vi "SC_schleife_20TVTI.vi"   [LabVIEW 2019]
uses:
  Monitors/Utility/Monitor Communication/Gustav/20TVTI_Control.ctl
  Global/Global Variables/global.vi
  Instrument_Setup.vi
  Global/Global Variables/Data_Display_global.vi
types:
  T1 = typedef "20TVTI_Cluster.ctl" = cluster{"Temperatur (K)":dbl, "Setpoint (K)":dbl, "Rate (K/min)":dbl, "Heater (%)":dbl, "NV (%)":dbl, "Heater Manual":bool, "NV Manual":bool, "Go to Set":bool, "Heater SP":dbl, "Valid?":bool, "Set Heater SP":bool, "Set NV SP":bool, "Heater (%) Display":dbl, "NV (%) Display":dbl, "NV Setpoint":dbl, "Change Heater Status":bool, "Change NV Status":bool, "Stop":bool, "Current T Setpoint":dbl, "Sweeping?":bool, "Sweep Mode":string, "Change Sweep Mode":bool}
  T2 = typedef "20TVTI_Control.ctl" = cluster{"Set VTI SP":bool, "Change NV Status":bool, "Set NV Setpoint":bool, "Change Heater Status":bool, "Set Heater Setpoint":bool, "Stop Sweep":bool, "Setpoint (K)":dbl, "Rate (K/min)":dbl, "Setpoint Heater":dbl, "Setpoint NV":dbl, "Change Sweep Mode":bool}
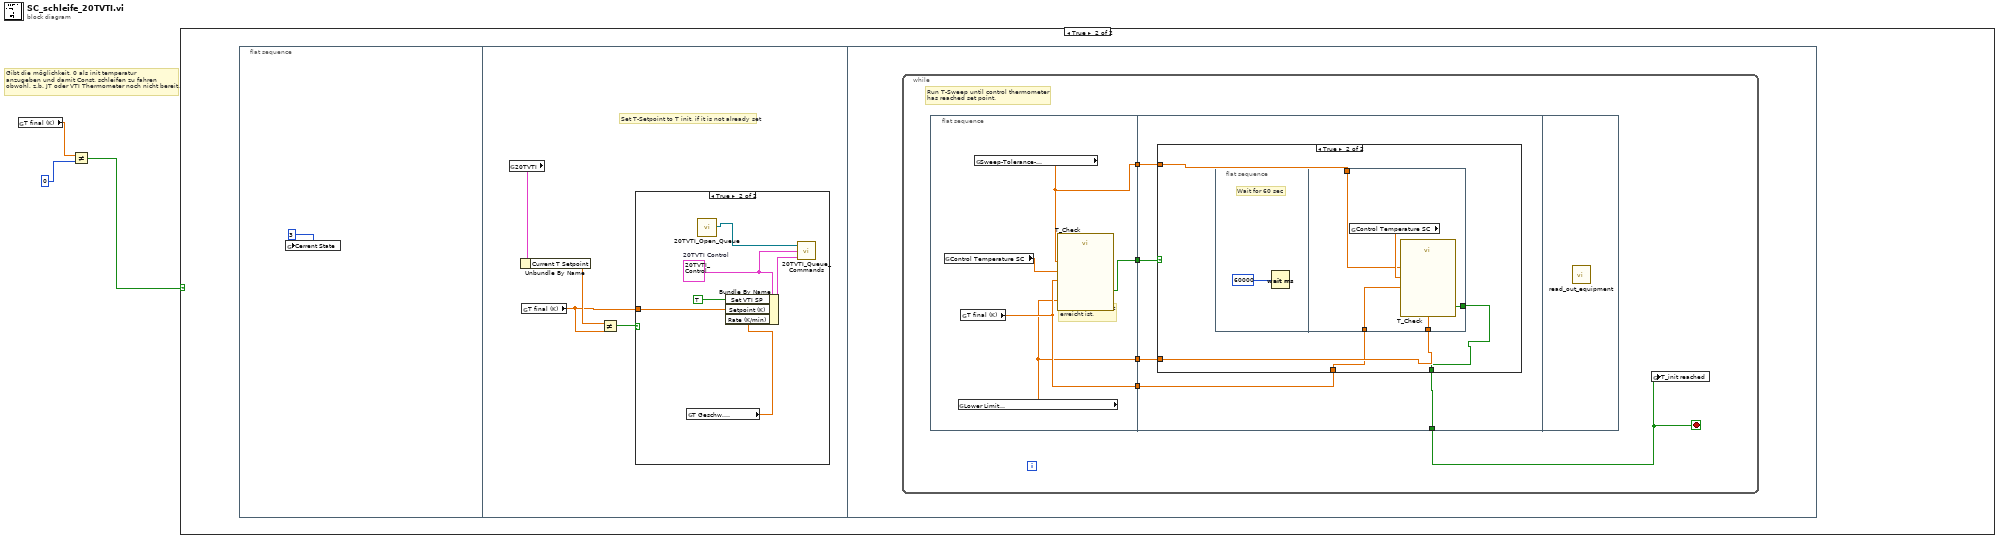
[diagram p0: block diagram]
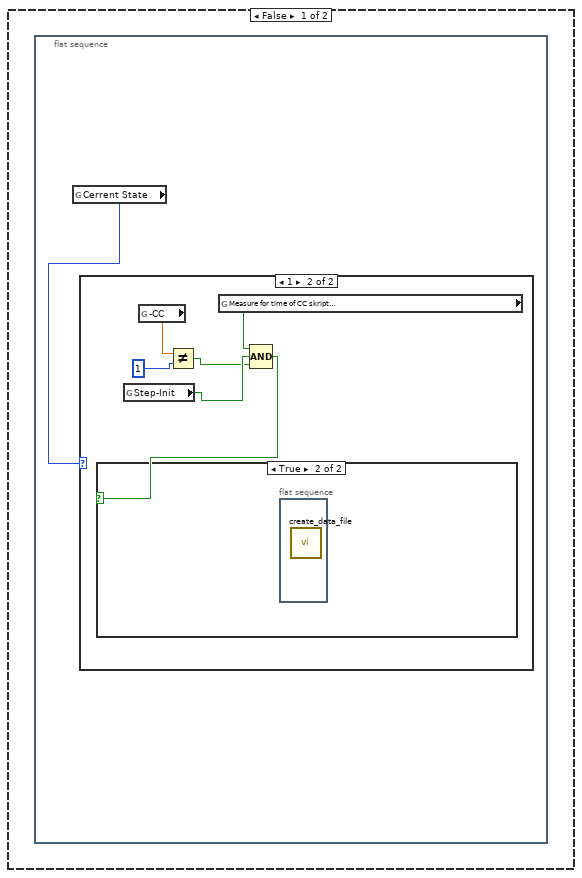
[diagram p2: hidden frame]
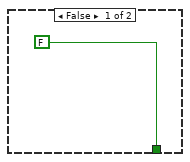
[diagram p6: hidden frame]
diagram:
  # "Gibt die möglichkeit, 0 als init temperatur \nanzugeben und damit Const. schleifen zu fahren\nobwohl, z.b. JT oder VTI Thermometer noch nicht bereit."
  n1 = global read "global.vi" "T final (K)"() -> (w3:dbl)
  n2 = Not Equal?(x=w3, y=0) -> (x != y?=w1:bool)
  n3 = case shown="True" w1 {
    frame False {
      n4 = flat-sequence {
        frame #0 {
          n5 = global read "global.vi" "Cerrent State"() -> (w4:i32)
          n6 = case shown="1" w4 {
            frame 0, Default {
            }
            frame 1 {
              n7 = global read "global.vi" "Step-Init"() -> (w8:bool)
              n8 = global read "global.vi" "-CC"() -> (w7:dbl)
              n9 = Not Equal?(x=w7, y=1) -> (x != y?=w5:bool)
              n10 = global read "Instrument_Setup.vi" "Measure for time of CC skript\nat each field step point"() -> (w10:bool)
              n11 = Compound Arithmetic op=AND(w10, w8, w5) -> (w9:bool)
              n12 = case shown="True" w9 {
                frame False {
                }
                frame True {
                  n13 = flat-sequence {
                    frame #0 {
                      n14 = call "create_data_file.vi"() -> ()  [unwired: 3 in]
                    }
                  }
                }
              }
            }
          }
        }
      }
    }
    frame True {
      n15 = flat-sequence {
        frame #0 {
          n16 = global write "global.vi" "Cerrent State"(3) -> ()
        }
        frame #1 {
          # "Set T-Setpoint to T init, if it is not already set"
          n17 = global read "Data_Display_global.vi" "20TVTI"() -> (w15:T1)
          n18 = Unbundle By Name(w15) -> ("Current T Setpoint"=w13:dbl)
          n19 = global read "global.vi" "T final (K)"() -> (w12:dbl)
          n20 = Not Equal?(x=w13, y=w12) -> (x != y?=w14:bool)
          n21 = case shown="True" w14 {
            tunnel: w12 -> [_ w20]
            frame False {
            }
            frame True {
              w16 = T2 {"Set VTI SP"=FALSE, "Change NV Status"=FALSE, "Set NV Setpoint"=FALSE, "Change Heater Status"=FALSE, "Set Heater Setpoint"=FALSE, "Stop Sweep"=FALSE, "Setpoint (K)"=0.0, "Rate (K/min)"=0.0, "Setpoint Heater"=0.0, "Setpoint NV"=0.0, "Change Sweep Mode"=FALSE}  # 20TVTI Control
              n22 = global read "global.vi" "T Geschw. \n(K/min)"() -> (w19:dbl)
              n23 = call "20TVTI_Open_Queue.vi"() -> ("queue out"=w18:refnum<queue>)  [unwired: 10 in, 1 out]
              n24 = Bundle By Name(cluster=w16, "Set VTI SP"=TRUE, "Setpoint (K)"=w20, "Rate (K/min)"=w19) -> (w17:T2)
              n25 = call "20TVTI_Queue_Commands.vi"("20TVTI Control"=w17, "Last Status"=w16, "20TVTI Queue"=w18) -> ()  [unwired: 1 out]
            }
          }
        }
        frame #2 {
          n26 = while {
            stop <- w26 stop-if-true
            # "Run T-Sweep until control thermometer\nhas reached set point."
            n27 = flat-sequence {
              tunnel: [w30] -> w25
              tunnel: [w29] -> w24
              tunnel: [w28] -> w23
              tunnel: [w27] -> w22
              tunnel: [w33] -> w26
              tunnel: w25 -> [w36]
              tunnel: w24 -> [w35]
              tunnel: w23 -> [w34]
              tunnel: w22 -> [w32]
              frame #0 {
                # "Check ob T_target\nerreicht ist."
                n28 = global read "Data_Display_global.vi" "Control Temperature SC"() -> (w31:dbl)
                n29 = global read "Instrument_Setup.vi" "Lower Limit\nSweep-Tolerance-\nTemperature (K)"() -> (w27:dbl)
                n30 = global read "global.vi" "T final (K)"() -> (w29:dbl)
                n31 = global read "Instrument_Setup.vi" "Sweep-Tolerance-\nTemperature (%)"() -> (w28:dbl)
                n32 = call "T_Check.vi"("Lower Limit Sweep\nTolerance (K)"=w27, "T_target (K)"=w29, "Sweep\nTolerance %"=w28, "T_in"=w31) -> ("= T target"=w30:bool)
              }
              frame #1 {
                n33 = case shown="True" w36 {
                  tunnel: w35 -> [_ w39]
                  tunnel: w34 -> [_ w41]
                  tunnel: [FALSE w38] -> w33
                  tunnel: w32 -> [_ w40]
                  frame False {
                  }
                  frame True {
                    n34 = flat-sequence {
                      tunnel: [w46] -> w38
                      tunnel: w39 -> [w45]
                      tunnel: w41 -> [w44]
                      tunnel: w40 -> [w43]
                      frame #0 {
                        # "Wait for 60 sec"
                        n35 = Wait (ms)(milliseconds to wait=60000) -> ()  [unwired: 1 out]
                      }
                      frame #1 {
                        n36 = global read "Data_Display_global.vi" "Control Temperature SC"() -> (w47:dbl)
                        n37 = call "T_Check.vi"("Lower Limit Sweep\nTolerance (K)"=w43, "T_target (K)"=w45, "Sweep\nTolerance %"=w44, "T_in"=w47) -> ("= T target"=w46:bool)
                      }
                    }
                  }
                }
              }
              frame #2 {
                n38 = call "read_out_equipment.vi"() -> ()  [unwired: 1 in]
              }
            }
            n39 = global write "Data_Display_global.vi" "T_init reached"(w26) -> ()
          }
        }
      }
    }
  }
